vi "cam0-测试夹角函数计算过程效果.vi"() -> ()   [LabVIEW 2015]
uses:
  <vilib>/vision/NI_Vision_Development_Module.lvlib
panel:
  in  "产品位 3":cluster{"X":sgl, "Y":sgl}
  in  "中心位 3":cluster{"X":sgl, "Y":sgl}
  in  "槽点位 3":cluster{"X":sgl, "Y":sgl}
  out "Angles (deg) 3":sgl[](array[numeric]) format="%.2f"
  in  "产品位 2":cluster{"X":sgl, "Y":sgl}
  in  "中心位 2":cluster{"X":sgl, "Y":sgl}
  in  "槽点位 2":cluster{"X":sgl, "Y":sgl}
  out "Angles (deg) 2":sgl[](array[numeric]) format="%.2f"
  out "Angles (deg)":sgl[](array[numeric]) format="%.2f"
  in  "槽点位":cluster{"X":sgl, "Y":sgl}
  in  "中心位":cluster{"X":sgl, "Y":sgl}
  in  "产品位":cluster{"X":sgl, "Y":sgl}
  # "数学的直角坐标系，非图像坐标系"
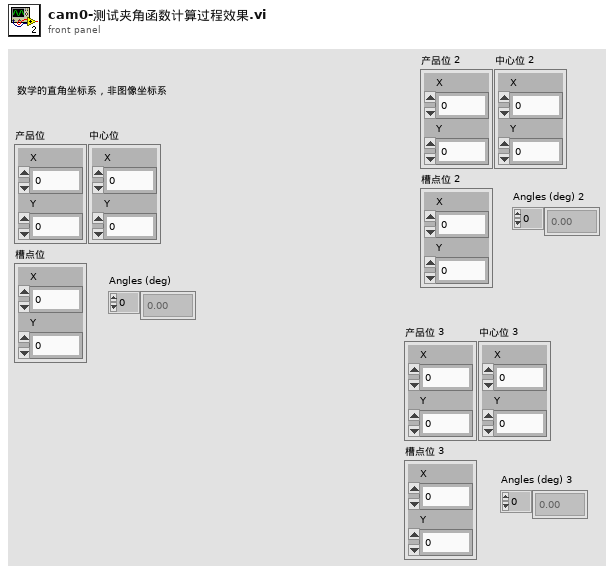
[diagram p1: front panel]
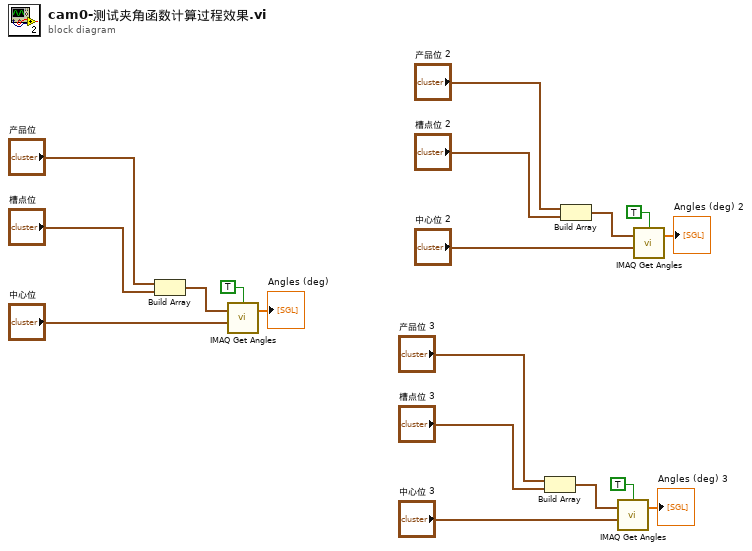
[diagram p0: block diagram]
diagram:
  n1 = Build Array("产品位", "槽点位") -> (w16:cluster{"X":sgl, "Y":sgl}[])
  n2 = call "IMAQ Get Angles"("Vertex"="中心位", "Points"=w16, "Use Vertex (No)"=TRUE) -> ("Angles (deg)"=→"Angles (deg)":sgl[])  [unwired: 2 in, 2 out]
  n3 = Build Array("产品位 3", "槽点位 3") -> (w4:cluster{"X":sgl, "Y":sgl}[])
  n4 = Build Array("产品位 2", "槽点位 2") -> (w9:cluster{"X":sgl, "Y":sgl}[])
  n5 = call "IMAQ Get Angles"("Vertex"="中心位 3", "Points"=w4, "Use Vertex (No)"=TRUE) -> ("Angles (deg)"=→"Angles (deg) 3":sgl[])  [unwired: 2 in, 2 out]
  n6 = call "IMAQ Get Angles"("Vertex"="中心位 2", "Points"=w9, "Use Vertex (No)"=TRUE) -> ("Angles (deg)"=→"Angles (deg) 2":sgl[])  [unwired: 2 in, 2 out]
